vi "Remove DC Offset.vi"(4 "Signal":dbl[](array[numeric])) -> (1 "Processed Signal":dbl[](array[numeric]))   [LabVIEW 2013]
uses:
  <vilib>/Analysis/baseanly.llb/Mean (DBL).vi
  <vilib>/Analysis/NI_AALBase.lvlib
panel:
  out "Processed Signal":dynamicdata(graph)
  out "Raw Signal":dynamicdata(graph)
  out "Standard Dev":dbl
  out "Arithmetic Mean":dbl
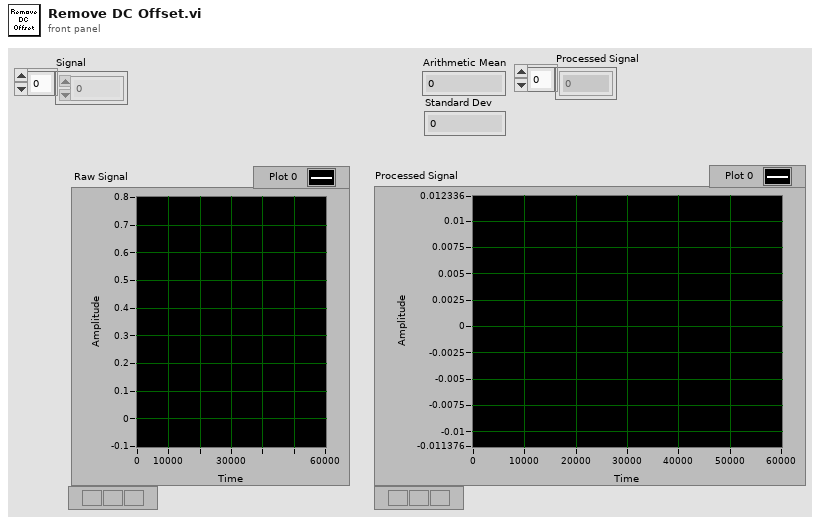
[diagram p1: front panel]
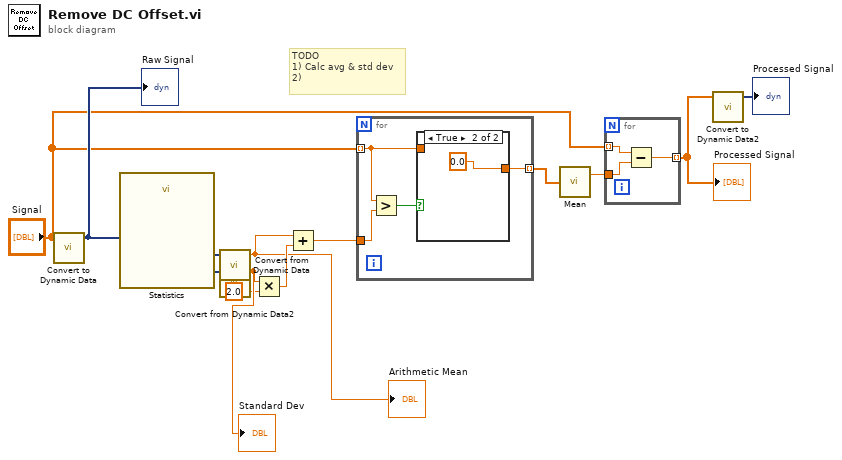
[diagram p0: block diagram]
diagram:
  # "TODO\n1) Calc avg & std dev\n2)"
  n1 = call "Convert to Dynamic Data"("Array"="Signal") -> ("Dynamic Data Type"=w13:dynamicdata)  [unwired: 3 in]
  "Raw Signal" <- w13
  n2 = call "Statistics"("Signals"=w13) -> ("Standard Dev"=w11:dynamicdata, "Arithmetic Mean"=w12:dynamicdata)  [unwired: 24 in, 1 out]
  n3 = call "Convert from Dynamic Data"("Dynamic Data Type"=w12) -> ("Scalar"=w7:dbl)  [unwired: 3 in]
  "Arithmetic Mean" <- w7
  n4 = call "Convert from Dynamic Data2"("Dynamic Data Type"=w11) -> ("Scalar"=w10:dbl)  [unwired: 3 in]
  "Standard Dev" <- w10
  n5 = Multiply(x=w10, y=2.0) -> (x*y=w8:dbl)
  n6 = Add(x=w7, y=w8) -> (x+y=w6:dbl)
  n7 = for {
    tunnel: "Signal" -> [w15] mode=indexing
    tunnel: w6 -> [w17]
    tunnel: [w14] -> w5 mode=indexing
    n8 = Greater?(x=w15, y=w17) -> (0:w16:bool)
    n9 = case shown="True" w16 {
      tunnel: w15 -> [w18 _]
      tunnel: [w18 0.0] -> w14
      frame False {
      }
      frame True {
      }
    }
  }
  n10 = call-poly <vilib>:"Mean.vi"("X"=w5) -> ("mean"=w4:dbl)  [unwired: 1 out]
  n11 = for {
    tunnel: "Signal" -> [w22] mode=indexing
    tunnel: w4 -> [w21]
    tunnel: [w20] -> w3 mode=indexing
    n12 = Subtract(x=w22, y=w21) -> (x-y=w20:dbl)
  }
  "Processed Signal" <- w3
  n13 = call "Convert to Dynamic Data2"("Array"=w3) -> ("Dynamic Data Type"=→"Processed Signal":dynamicdata)  [unwired: 3 in]
